vi "Serial Terminal.vi"() -> ()   [LabVIEW 2021]
doc: "This VI example allows the user to send the SCIP commands to the instrument U1282A. The VI behaves like a serial terminal, where the user use the Read and Write buttons to send and receive the information of the instrument."
uses:
  <vilib>/Utility/error.llb/Error Cluster From Error Code.vi
  <vilib>/ErrorRing/Error Ring.xnode
  Keysight U1282A.lvlib
panel:
  in  "Serial Configuration":T1={"Baud Rate"=enum."9600", "Timeout"=10000, "Stop Bits"=10, "Flow Control"=enum."None", "Parity"=0}
  in  "Exit":bool
  in  "Count":i32=50 caption="Auto hold mode count (TRIG:REF:COUN)"
  in  "SCIP Command":string(combo)="*IDN?"
  out "Reading":string
  out "Bytes at port":u32
  in  "VISA resource name":refnum<visa-resource-name>="Keysight_U1282A"
  in  "Read":bool
  in  "Write":bool
  out "error out":errorcluster
  in  "error in":errorcluster
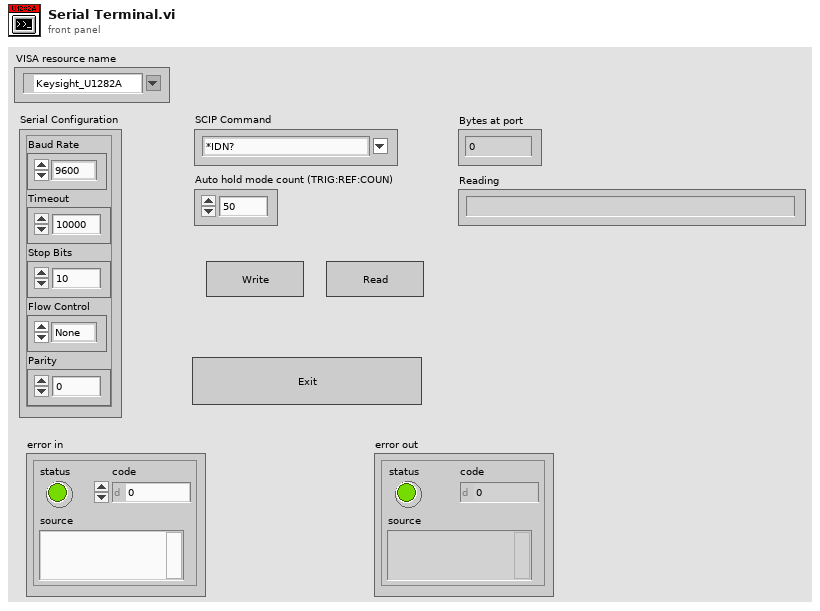
[diagram p1: front panel]
types:
  T1 = cluster{"Baud Rate":enum16{"1200", "2400", "4800", "9600", "19200", "38400", "57600", "115200"}, "Timeout":u32, "Stop Bits":u16, "Flow Control":enum16{"None", "XON / XOFF", "RTS / CTS", "DTR / DSR"}, "Parity":u16}
  T2 = cluster{"VISA resource name":refnum<visa-resource-name>, "Serial Configuration":cluster{"Baud Rate":enum16{"1200", "2400", "4800", "9600", "19200", "38400", "57600", "115200"}, "Timeout":u32, "Stop Bits":u16, "Flow Control":enum16{"None", "XON / XOFF", "RTS / CTS", "DTR / DSR"}, "Parity":u16}, "Value":string, "Reading":string, "Bytes at port":u32}
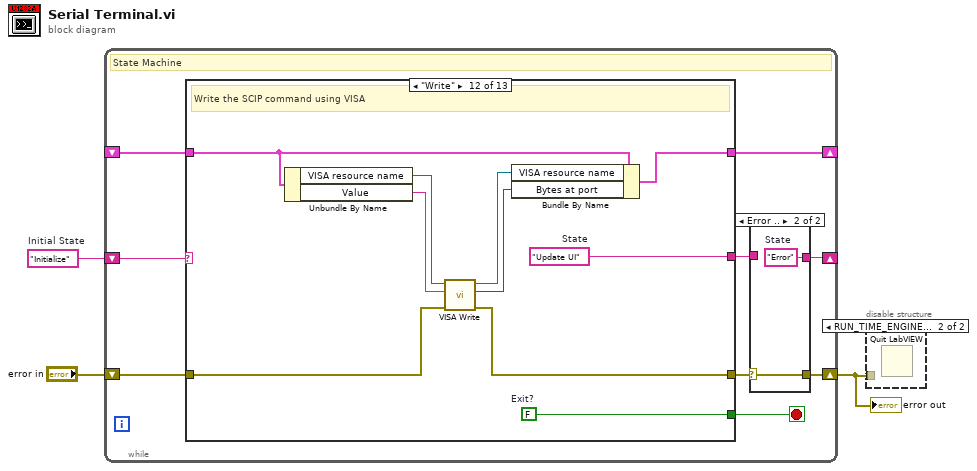
[diagram p0: block diagram]
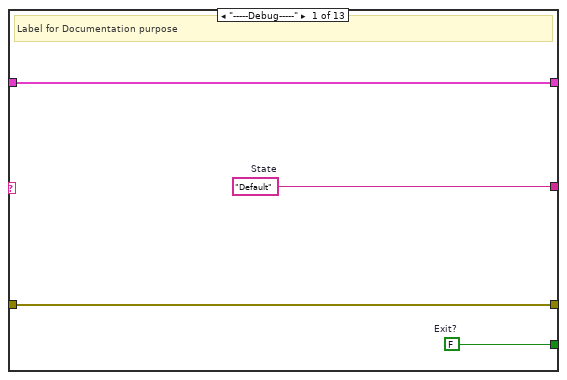
[diagram p2: hidden frame]
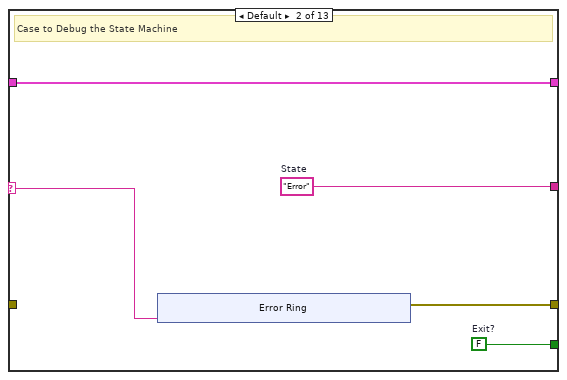
[diagram p3: hidden frame]
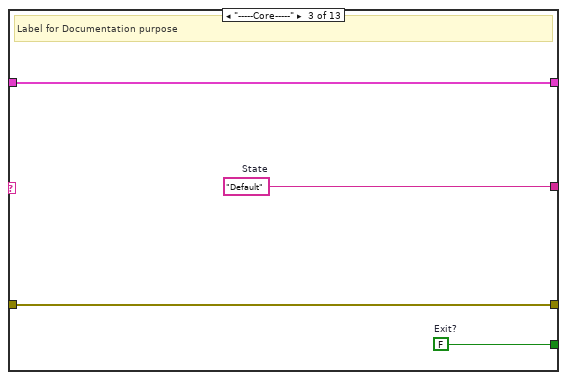
[diagram p4: hidden frame]
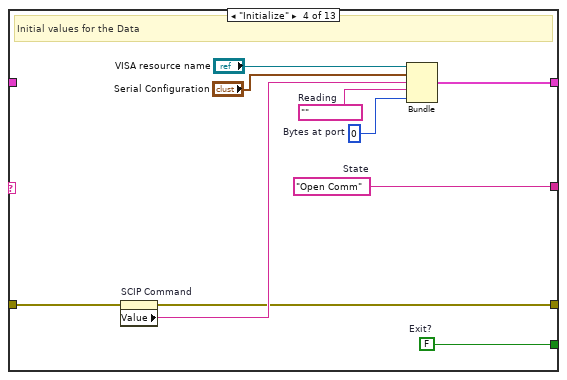
[diagram p5: hidden frame]
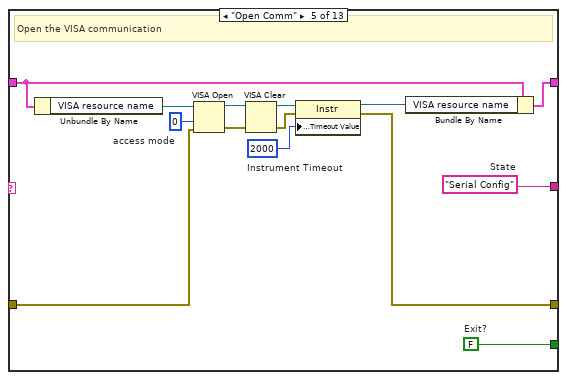
[diagram p6: hidden frame]
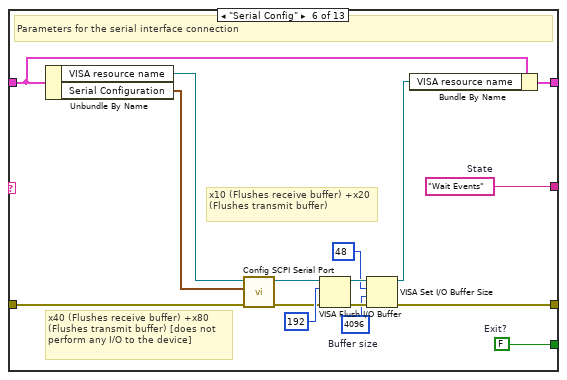
[diagram p7: hidden frame]
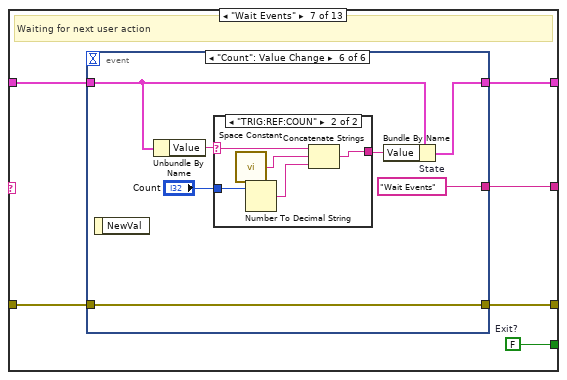
[diagram p8: hidden frame]
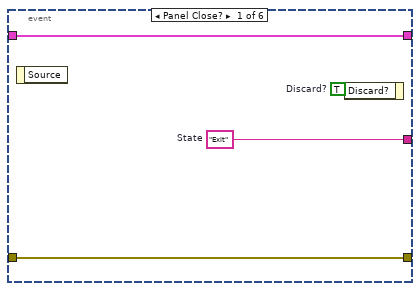
[diagram p9: hidden frame]
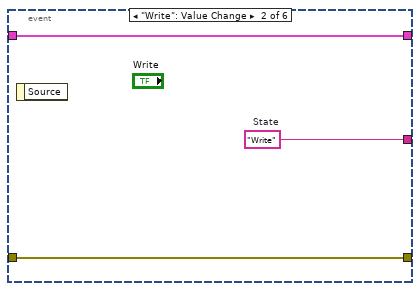
[diagram p10: hidden frame]
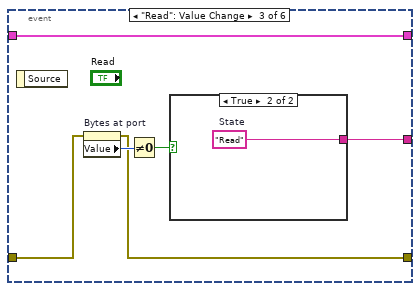
[diagram p11: hidden frame]
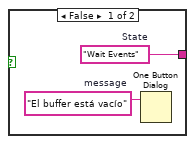
[diagram p12: hidden frame]
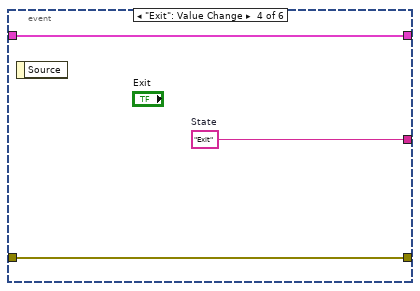
[diagram p13: hidden frame]
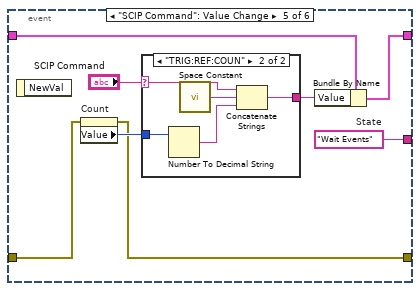
[diagram p14: hidden frame]
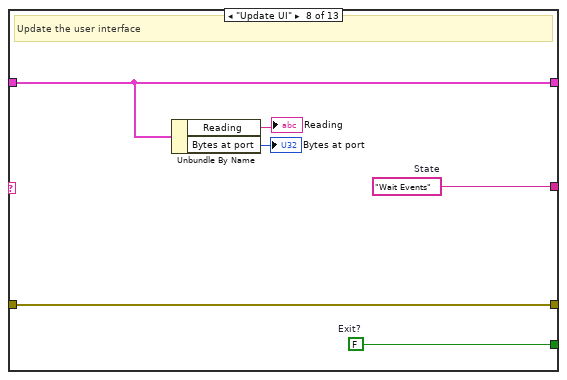
[diagram p17: hidden frame]
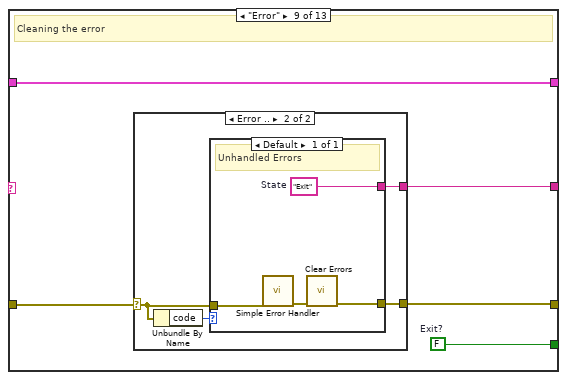
[diagram p18: hidden frame]
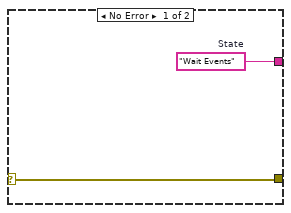
[diagram p19: hidden frame]
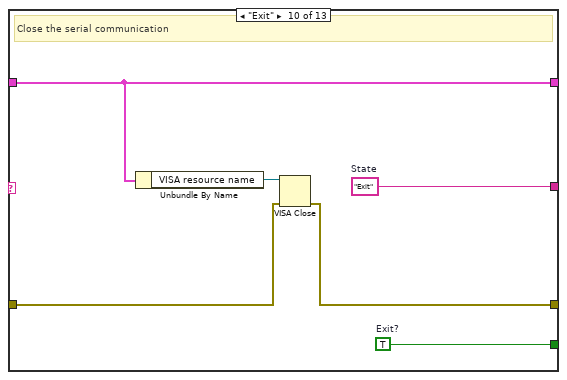
[diagram p20: hidden frame]
diagram:
  w3 = "Initialize"  # Initial State
  n1 = while {
    shift-right: [w11] -> _
    shift-left: w3 -> [w12]
    shift-right: [w9] -> w1
    shift-left: "error in" -> [w8]
    shift-right: [w6] -> _
    shift-left: _ -> [w5]
    stop <- w7 stop-if-true
    # "State Machine"
    n2 = case shown="\"Write\"" w12 {
      selector: w12 -> [_ w20 _ _ _ _ _ _ _ _ _ _ _]
      tunnel: [w16 w21 w32 w40 w43 w66 w77 w127 w133 w151 w155 w165 w175] -> w4
      tunnel: [w15 w19 w31 w35 w51 w69 w76 w126 w134 w148 w153 w162 w171] -> w10
      tunnel: w8 -> [w15 _ w31 w36 w44 w63 w78 w126 w135 w149 w153 w156 w172]
      tunnel: [w13 w17 w29 w34 w50 w62 w75 w125 w131 w150 w152 w157 w167] -> w7
      tunnel: [w14 w18 w30 w41 w47 w57 w74 w130 w132 w146 w154 w164 w176] -> w6
      tunnel: w5 -> [w14 w18 w30 _ w45 w58 w73 w130 w132 w146 w154 w163 w166]
      frame "-----Debug-----" {
        w13 = FALSE  # Exit?
        w16 = "Default"  # State
        # "Label for Documentation purpose"
      }
      frame Default {
        w17 = FALSE  # Exit?
        w21 = "Error"  # State
        # "Case to Debug the State Machine"
        n3 = xnode "Error Ring"("parameter 0"=w20) -> ("error out"=w19:errorcluster)
      }
      frame "-----Core-----" {
        w29 = FALSE  # Exit?
        w32 = "Default"  # State
        # "Label for Documentation purpose"
      }
      frame "Initialize" {
        w34 = FALSE  # Exit?
        w38 = u32 0  # Bytes at port
        w39 = ""  # Reading
        w40 = "Open Comm"  # State
        # "Initial values for the Data"
        n4 = property on="SCIP Command" class="CmbBox"(error in=w36) -> (error out=w35:errorcluster, "Value"=w37:string)  [unwired: 1 in, 1 out]
        n5 = Bundle("VISA resource name"="VISA resource name", "Serial Configuration"="Serial Configuration", "Value"=w37, "Reading"=w39, "Bytes at port"=w38) -> (w41:T2)  [unwired: 1 in]
      }
      frame "Open Comm" {
        w50 = FALSE  # Exit?
        w43 = "Serial Config"  # State
        w53 = u32 0  # access mode
        w52 = u32 2000  # Instrument Timeout
        # "Open the VISA communication"
        n6 = Unbundle By Name(w45) -> ("VISA resource name"=w48:refnum<visa-resource-name>)
        n7 = VISA Open(access mode=w53, error in (no error)=w44, VISA resource name=w48) -> (VISA resource name=w49:refnum<visa-resource-name>, error out=w56:errorcluster)  [unwired: 2 in]
        n8 = VISA Clear(VISA resource name=w49, error in (no error)=w56) -> (VISA resource name out=w55:refnum<visa-resource-name>, error out=w54:errorcluster)
        n9 = property class="Instr"(reference=w55, error in=w54, "General Settings:Timeout Value"=w52) -> (reference out=w46:refnum<visa-resource-name>, error out=w51:errorcluster)
        n10 = Bundle By Name(cluster=w45, "VISA resource name"=w46) -> (w47:T2)
      }
      frame "Serial Config" {
        w62 = FALSE  # Exit?
        w66 = "Wait Events"  # State
        w70 = u32 4096  # Buffer size
        # "x40 (Flushes receive buffer) +x80 (Flushes transmit buffer) [does not perform any I/O to the device]"
        # "x10 (Flushes receive buffer) +x20 (Flushes transmit buffer)"
        # "Parameters for the serial interface connection"
        n11 = Unbundle By Name(w58) -> ("VISA resource name"=w59:refnum<visa-resource-name>, "Serial Configuration"=w61:T1)
        n12 = call "Config SCPI Serial Port.vi"("error in"=w63, "Settings"=w61, "VISA Refnum in"=w59) -> ("error out"=w64:errorcluster, "VISA Refnum out"=w65:refnum<visa-resource-name>)  [unwired: 7 in]
        n13 = VISA Flush I/O Buffer(VISA resource name=w65, mask (16)=u16 192, error in (no error)=w64) -> (VISA resource name out=w72:refnum<visa-resource-name>, error out=w71:errorcluster)
        n14 = VISA Set I/O Buffer Size(VISA resource name=w72, mask (16)=u16 48, size (4096)=w70, error in (no error)=w71) -> (VISA resource name out=w60:refnum<visa-resource-name>, error out=w69:errorcluster)
        n15 = Bundle By Name(cluster=w58, "VISA resource name"=w60) -> (w57:T2)
      }
      frame "Wait Events" {
        w75 = FALSE  # Exit?
        # "Waiting for next user action"
        n16 = event shown="[5] \"Count\": Value Change" {
          selector: _ -> [_ _ _ _ _ _]
          dyn-events: _ -> [_ _ _ _ _ _]
          timeout: _ -> [_ _ _ _ _ _]
          tunnel: w78 -> [w82 w83 w88 w95 w99 w115]
          tunnel: [w82 w83 w87 w95 w98 w115] -> w76
          tunnel: [w80 w84 w89 w96 w103 w114] -> w77
          tunnel: w73 -> [w79 w85 w86 w97 w105 w117]
          tunnel: [w79 w85 w86 w97 w104 w116] -> w74
          event Panel Close? {
            w80 = "Exit"  # State
            w81 = TRUE  # Discard?
            n17 = event-data() -> ()  [unwired: 1 in, 1 out]
            n18 = event-data("Discard?"=w81) -> ()  [unwired: 1 in, 1 out]
          }
          event "Write": Value Change {
            w84 = "Write"  # State
            n19 = event-data() -> ()  [unwired: 1 in, 1 out]
          }
          event "Read": Value Change {
            n20 = event-data() -> ()  [unwired: 1 in, 1 out]
            n21 = property on="Bytes at port" class="DigNum (strict)"(error in=w88) -> (error out=w87:errorcluster, "Value"=w91:u32)  [unwired: 1 in, 1 out]
            n22 = Not Equal To 0?(x=w91) -> (x != 0?=w90:bool)
            n23 = case shown="True" w90 {
              tunnel: [w93 w94] -> w89
              frame False {
                w92 = "El buffer está vacío"  # message
                w93 = "Wait Events"  # State
                n24 = One Button Dialog(message=w92) -> ()  [unwired: 1 in, 1 out]
              }
              frame True {
                w94 = "Read"  # State
              }
            }
          }
          event "Exit": Value Change {
            w96 = "Exit"  # State
            n25 = event-data() -> ()  [unwired: 1 in, 1 out]
          }
          event "SCIP Command": Value Change {
            w103 = "Wait Events"  # State
            n26 = event-data() -> ()  [unwired: 1 in, 1 out]
            n27 = property on="Count" class="DigNum (strict)"(error in=w99) -> (error out=w98:errorcluster, "Value"=w101:i32)  [unwired: 1 in, 1 out]
            n28 = case shown="\"TRIG:REF:COUN\"" "SCIP Command" {
              selector: "SCIP Command" -> [w106 w110]
              tunnel: w101 -> [_ w111]
              tunnel: [w106 w107] -> w100
              frame Default {
              }
              frame "TRIG:REF:COUN" {
                n29 = Number To Decimal String(number=w111) -> (decimal integer string=w108:string)  [unwired: 1 in]
                n30 = call <vilib>:"Space Constant.vi"() -> ("String"=w109:string)
                n31 = Concatenate Strings(w110, w109, w108) -> (w107:string)
              }
            }
            n32 = Bundle By Name(cluster=w105, "Value"=w100) -> (w104:T2)
          }
          event "Count": Value Change {
            w114 = "Wait Events"  # State
            n33 = event-data() -> ()  [unwired: 1 in, 1 out]
            n34 = Unbundle By Name(w117) -> ("Value"=w112:string)
            n35 = case shown="\"TRIG:REF:COUN\"" w112 {
              selector: w112 -> [w119 w120]
              tunnel: "Count" -> [_ w124]
              tunnel: [w119 w121] -> w113
              frame Default {
              }
              frame "TRIG:REF:COUN" {
                n36 = call <vilib>:"Space Constant.vi"() -> ("String"=w123:string)
                n37 = Number To Decimal String(number=w124) -> (decimal integer string=w122:string)  [unwired: 1 in]
                n38 = Concatenate Strings(w120, w123, w122) -> (w121:string)
              }
            }
            n39 = Bundle By Name(cluster=w117, "Value"=w113) -> (w116:T2)
          }
        }
      }
      frame "Update UI" {
        w125 = FALSE  # Exit?
        w127 = "Wait Events"  # State
        # "Update the user interface"
        n40 = Unbundle By Name(w130) -> ("Reading"=→"Reading":string, "Bytes at port"=→"Bytes at port":u32)
      }
      frame "Error" {
        w131 = FALSE  # Exit?
        # "Cleaning the error"
        n41 = case shown="Error .." w135 {
          selector: w135 -> [w136 w138]
          tunnel: [w136 w140] -> w134
          tunnel: [w137 w139] -> w133
          frame No Error {
            w137 = "Wait Events"  # State
          }
          frame Error {
            n42 = Unbundle By Name(w138) -> ("code"=w141:i32)
            n43 = case shown="Default" w141 {
              tunnel: w138 -> [w143]
              tunnel: [w144] -> w140
              tunnel: [w142] -> w139
              frame Default {
                w142 = "Exit"  # State
                # "Unhandled Errors"
                n44 = call <vilib>:"Simple Error Handler.vi"("error in (no error)"=w143) -> ("error out"=w145:errorcluster)  [unwired: 4 in, 4 out]
                n45 = call <vilib>:"Clear Errors.vi"("error in (no error)"=w145) -> ("error out"=w144:errorcluster)  [unwired: 5 in, 1 out]
              }
            }
          }
        }
      }
      frame "Exit" {
        w150 = TRUE  # Exit?
        w151 = "Exit"  # State
        # "Close the serial communication"
        n46 = Unbundle By Name(w146) -> ("VISA resource name"=w147:refnum<visa-resource-name>)
        n47 = VISA Close(VISA resource name=w147, error in (no error)=w149) -> (error out=w148:errorcluster)
      }
      frame "-----States-----" {
        w152 = FALSE  # Exit?
        w155 = "Default"  # State
        # "Label for Documentation purpose"
      }
      frame "Write" {
        w157 = FALSE  # Exit?
        w165 = "Update UI"  # State
        # "Write the SCIP command using VISA"
        n48 = Unbundle By Name(w163) -> ("VISA resource name"=w160:refnum<visa-resource-name>, "Value"=w159:string)
        n49 = call "VISA Write.vi"("error in"=w156, "SCPI command"=w159, "VISA resource in"=w160) -> ("error out"=w162:errorcluster, "Bytes at Port out"=w158:u32, "VISA resource out"=w161:refnum<visa-resource-name>)  [unwired: 6 in]
        n50 = Bundle By Name(cluster=w163, "VISA resource name"=w161, "Bytes at port"=w158) -> (w164:T2)
      }
      frame "Read" {
        w167 = FALSE  # Exit?
        w175 = "Update UI"  # State
        # "Read the SCIP command using VISA"
        n51 = Unbundle By Name(w166) -> ("VISA resource name"=w174:refnum<visa-resource-name>, "Bytes at port"=w173:u32)
        n52 = call "VISA Read.vi"("error in"=w172, "Bytes at Port in"=w173, "VISA resource in"=w174) -> ("error out"=w171:errorcluster, "Reading"=w168:string, "Bytes at Port out"=w169:u32, "VISA resource out"=w170:refnum<visa-resource-name>)  [unwired: 5 in]
        n53 = Bundle By Name(cluster=w166, "VISA resource name"=w170, "Bytes at port"=w169, "Reading"=w168) -> (w176:T2)
      }
    }
    n54 = case shown="Error .." w10 {
      selector: w10 -> [w177 w179]
      tunnel: w4 -> [w178 _]
      tunnel: [w178 w180] -> w11
      tunnel: [w177 w179] -> w9
      frame No Error {
      }
      frame Error {
        w180 = "Error"  # State
      }
    }
  }
  "error out" <- w1
  n55 = disable-structure shown="RUN_TIME_ENGINE==True" {
    disable-tunnel: w1 -> [_ _]
    frame condition #0 (active) {
    }
    frame condition #1 {
      n56 = Quit LabVIEW() -> ()  [unwired: 1 in]
    }
  }
